vi "Set Multi.vi"(0 "Display State In":T1, 5 "Value":i16, 7 "First":bool, 9 "Container State":T2, 11 "error in (no error)":errorcluster) -> (4 "Display State Out":T1, 6 "mixed":bool, 15 "error out":errorcluster)   [LabVIEW 2015, in "KRing.xctl"]
uses:
  KRing.xctl
  <vilib>/_xctls/Container State.ctl
  State.ctl
  <vilib>/_xctls/XControlSupport.lvlib
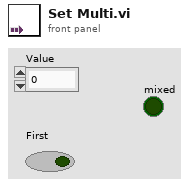
[diagram p1: front panel]
types:
  T1 = typedef "KRing.xctl/State.ctl" = cluster{"mixed":bool, "Value":i16, "Ring":refnum<vi>}
  T2 = typedef "XControlSupport.lvlib/Container State.ctl" = cluster{"Indicator?":bool, "Run Mode?":bool, " Refnum":refnum<vi>}
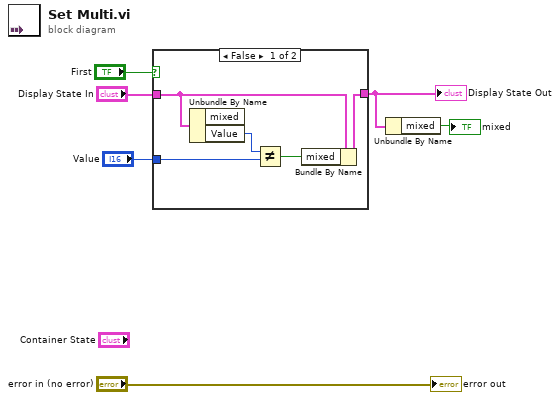
[diagram p0: block diagram]
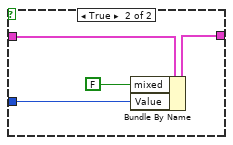
[diagram p2: hidden frame]
diagram:
  n1 = case shown="False" "First" {
    tunnel: "Display State In" -> [w11 w15]
    tunnel: [w8 w14] -> w2
    tunnel: "Value" -> [w9 w12]
    frame False {
      n2 = Unbundle By Name(w11) -> ("Value"=w10:i16)  [unwired: 1 out]
      n3 = Not Equal?(x=w10, y=w9) -> (x != y?=w7:bool)
      n4 = Bundle By Name(cluster=w11, "mixed"=w7) -> (w8:T1)
    }
    frame True {
      n5 = Bundle By Name(cluster=w15, "mixed"=FALSE, "Value"=w12) -> (w14:T1)
    }
  }
  "Display State Out" <- w2
  n6 = Unbundle By Name(w2) -> ("mixed"=→"mixed":bool)
  "error out" <- "error in (no error)"
